vi "myRI0-1900.vi"() -> (0 "myRIO-1900":T1={"DI Channels"=[0, 1, 2, 3, 4, 5, 6, 7, 8, 9, 10, 11, 12, 13, 14, 15, 16, 17, 18, 19, 20, 21, 22, 23, 24, 25, 26, 27, 28, 29, 30, 31, 32, 33, 34, 35, 36, 37, 38, 39], "DO Channels"=[0, 1, 2, 3, 4, 5, 6, 7, 8, 9, 10, 11, 12, 13, 14, 15, 16, 17, 18, 19, 20, 21, 22, 23, 24, 25, 26, 27, 28, 29, 30, 31, 32, 33, 34, 35, 36, 37, 38, 39], "AI"=[0, 1, 2, 3, 4, 5, 6, 7, 8, 9, 10, 11], "AO"=[0, 1, 2, 3, 4, 5, 6, 7], "PWM"=[0, 1, 2, 3, 4, 5, 6, 7], "QE"=[0, 1], "UART"=[0, 1], "I2C 2"=[0, 1], "SPI"=[0, 1], "CAN"=[], "AI Ref (V)"=5.0, "Firmware Program Interfaces"=[enum."N/A"], "Firmware Versions"=[], "Name"="myRIO-1900", "AO Resolution (Bits)"=0, "AO Ref (V)"=0.0})   [LabVIEW 2013, in "LVH-LINX.lvlib"]
doc: "I/O description of the NI myRIO-1900."
uses:
  <vilib>/LabVIEW Hacker/LINX/LVH-LINX.lvlib
  <vilib>/LabVIEW Hacker/LINX/Private/Type Defs/Devices/Generic Device.ctl
  <vilib>/LabVIEW Hacker/LINX/Private/Type Defs/Firmware Version.ctl
  <vilib>/LabVIEW Hacker/LINX/Private/Device/Type Defs/Firmware Interface.ctl
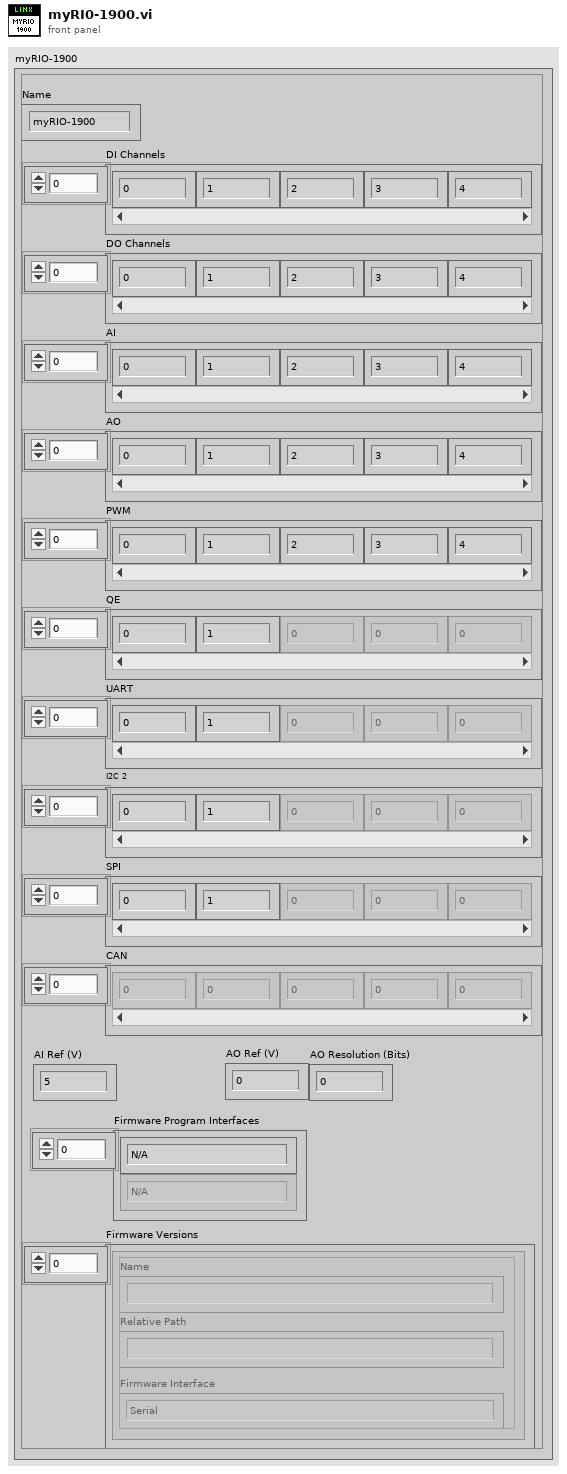
[diagram p1: front panel]
types:
  T1 = typedef "LVH-LINX.lvlib/Generic Device.ctl" = cluster{"DI Channels":u8[], "DO Channels":u8[], "AI":u8[], "AO":u8[], "PWM":u8[], "QE":u8[], "UART":u8[], "I2C 2":u8[], "SPI":u8[], "CAN":u8[], "AI Ref (V)":dbl, "Firmware Program Interfaces":enum16{"N/A", "Serial / USB", "USB", "TCP"}[], "Firmware Versions":T2[], "Name":string, "AO Resolution (Bits)":u8, "AO Ref (V)":dbl}
  T2 = typedef "LVH-LINX.lvlib/Firmware Version.ctl" = cluster{"Name":string, "Relative Path":string, "Firmware Interface":T3}
  T3 = typedef "LVH-LINX.lvlib/Firmware Interface.ctl" = enum32{"Serial ", "Ethernet", "WIFI"}
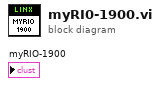
[diagram p0: block diagram]
diagram:
